vi "WPI_DashboardLog file path.vi"(11 "Time Date String":string) -> (3 "appended path":path)   [LabVIEW 2025]
uses:
  <vilib>/Utility/sysdir.llb/System Directory Type.ctl
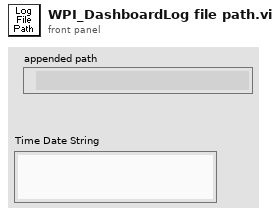
[diagram p1: front panel]
types:
  T1 = typedef "System Directory Type.ctl" = i32
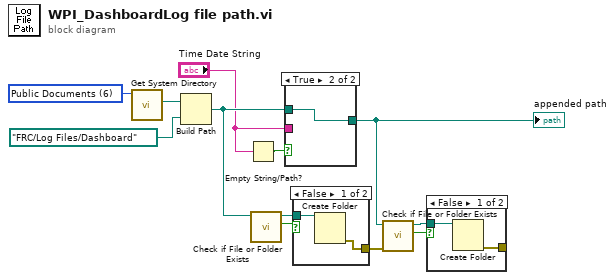
[diagram p0: block diagram]
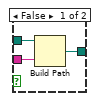
[diagram p2: hidden frame]
diagram:
  w12 = T1 6 items=["User Home"=0, "User Desktop"=1, "User Documents"=2, "User Application Data"=3, "User Preferences"=4, "User Temporary"=5, "Public Documents"=6, "Public Application Data"=7, "Public Preferences"=8, "Public Cache"=13, "System Core Libraries"=9, "System Installed Libraries"=10, "Application Files"=11, "Boot Volume Root"=12] ("system directory type")
  n1 = call <vilib>:"Get System Directory.vi"("system directory type"=w12) -> ("system directory"=w11:path)  [unwired: 10 in]
  n2 = Build Path(base path=w11, name or relative path=path "FRC/Log Files/Dashboard") -> (appended path=w7:path)
  n3 = Empty String/Path?(string/path="Time Date String") -> (empty?=w1:bool)
  n4 = call <vilib>:"Check if File or Folder Exists.vi"("path"=w7) -> ("file or folder exists?"=w9:bool, "dup path"=w8:path)  [unwired: 8 in, 1 out]
  n5 = case shown="True" w1 {
    tunnel: w7 -> [w15 w16]
    tunnel: "Time Date String" -> [w14 _]
    tunnel: [w13 w16] -> w4
    frame False {
      n6 = Build Path(base path=w15, name or relative path=w14) -> (appended path=w13:path)
    }
    frame True {
    }
  }
  "appended path" <- w4
  n7 = case shown="False" w9 {
    tunnel: w8 -> [w18 _]
    tunnel: [w17 _] -> w5
    frame False {
      n8 = Create Folder(path (use dialog)=w18) -> (error out=w17:errorcluster)  [unwired: 2 in, 2 out]
    }
    frame True {
    }
  }
  n9 = call <vilib>:"Check if File or Folder Exists.vi"("error in (no error)"=w5, "path"=w4) -> ("file or folder exists?"=w6:bool, "dup path"=w3:path)  [unwired: 7 in, 1 out]
  n10 = case shown="False" w6 {
    tunnel: w3 -> [w20 _]
    tunnel: [w19 _] -> _
    frame False {
      n11 = Create Folder(path (use dialog)=w20) -> (error out=w19:errorcluster)  [unwired: 2 in, 2 out]
    }
    frame True {
    }
  }
